vi "REFPROP2dll_Test.vi"(8 "error in (no error)":errorcluster) -> (0 "error out":errorcluster, 3 "Passed?":bool)   [LabVIEW 2016]
panel:
  out "Inputs":T1
  out "Outputs":T2 {"Output" format="%#_9g"}
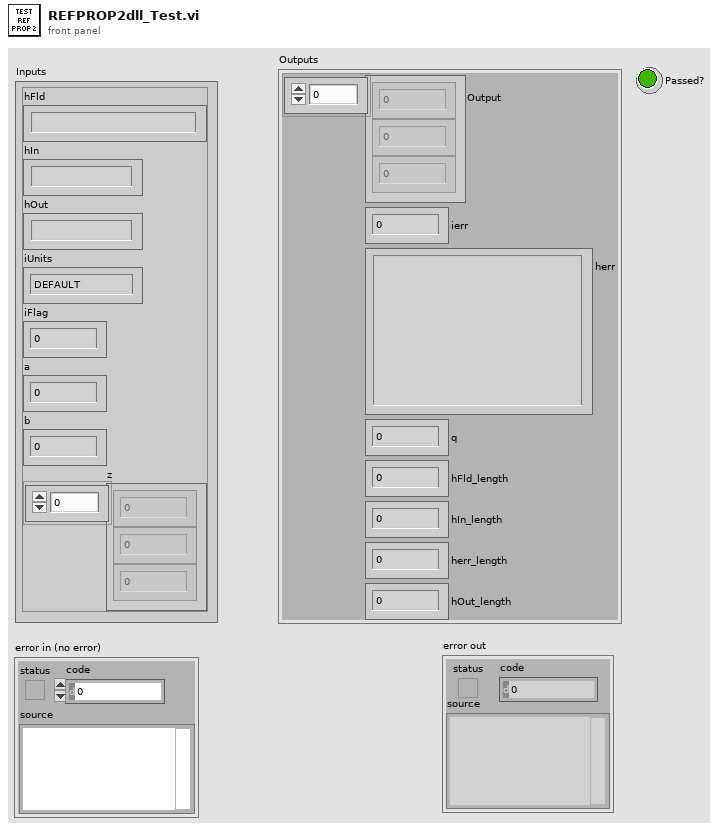
[diagram p1: front panel]
types:
  T1 = cluster{"hFld":string, "hIn":string, "hOut":string, "iUnits":enum32{"DEFAULT", "MOLE SI", "MASS SI", "SI WITH C"}, "iFlag":i32, "a":dbl, "b":dbl, "z":dbl[]}
  T2 = cluster{"Output":dbl[], "ierr":i32, "herr":string, "q":dbl, "hFld_length":i32, "hIn_length":i32, "hOut_length":i32, "herr_length":i32}
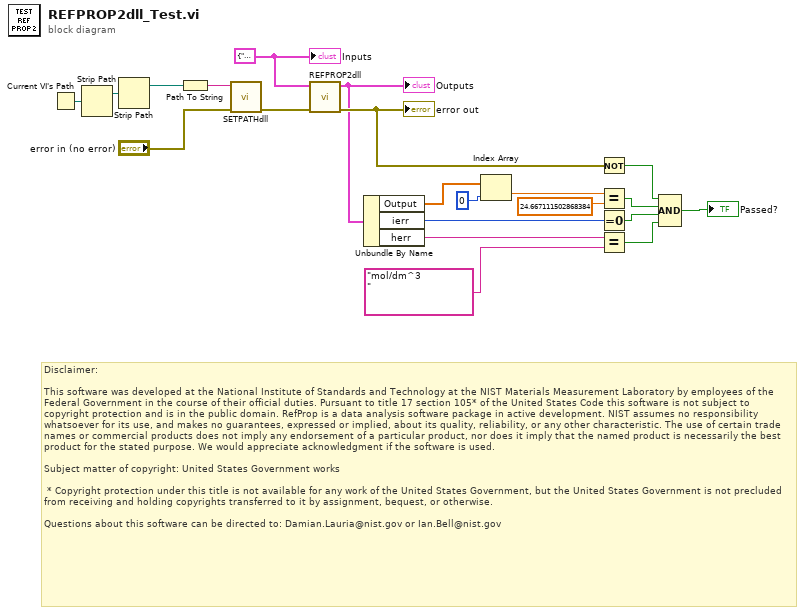
[diagram p0: block diagram]
diagram:
  w16 = T1 {"hFld"="Methane * Ethane", "hIn"="TQ", "hOut"="D", "iUnits"=enum."DEFAULT", "iFlag"=0, "a"=80.0, "b"=0.0, "z"=[0.4, 0.6]} ("Inputs")
  # "Disclaimer:\n\nThis software was developed at the National Institute of Standards and Technology at the NIST Materials Measurement Laboratory by employees of the Federal Government in the course of their official duties. Pursuant to title 17 section 105* of the United States Code this software is not subject to copyright protection and is in the public domain. RefProp is a data analysis software package in active development. NIST assumes no responsibility whatsoever for its use, and makes no guarantees, expressed or implied, about its quality, reliability, or any other characteristic. The use of certain trade names or commercial products does not imply any endorsement of a particular product, nor does it imply that the named product is necessarily the best product for the stated purpose. We would appreciate acknowledgment if the software is used.\n \nSubject matter of copyright: United States Government works\n  \n * Copyright protection under this title is not available for any work of the United States Government, but the United States Government is not precluded from receiving and holding copyrights transferred to it by assignment, bequest, or otherwise.\n\nQuestions about this software can be directed to: Damian.Lauria@nist.gov or Ian.Bell@nist.gov"
  n1 = Current VI's Path() -> (path=w21:path)
  n2 = Strip Path(path=w21) -> (stripped path=w20:path)  [unwired: 1 out]
  n3 = Strip Path(path=w20) -> (stripped path=w19:path)  [unwired: 1 out]
  n4 = Path To String(path=w19) -> (string=w18:string)
  n5 = call "SETPATHdll.vi"("error in (no error)"="error in (no error)", "hpath"=w18) -> ("error out"=w15:errorcluster)  [unwired: 7 in, 2 out]
  n6 = call "REFPROP2dll.vi"("error in (no error)"=w15, "Inputs"=w16) -> ("error out"=w14:errorcluster, "Outputs"=w13:T2)  [unwired: 8 in]
  "error out" <- w14
  "Outputs" <- w13
  n7 = Unbundle By Name(w13) -> ("Output"=w11:dbl[], "ierr"=w12:i32, "herr"=w7:string)
  n8 = Index Array(array=w11, index=0) -> (element=w10:dbl)
  n9 = Not(x=w14) -> (.not. x?=w5:bool)
  n10 = Equal?(x=w10, y=24.667111502868384 ("element")) -> (x = y?=w4:bool)
  n11 = Equal To 0?(x=w12) -> (x = 0?=w3:bool)
  n12 = Equal?(x=w7, y="mol/dm^3                                                                                                                                                                                                                                                      ") -> (x = y?=w2:bool)
  n13 = Compound Arithmetic op=AND(w5, w4, w3, w2) -> (→"Passed?":bool)
  "Inputs" <- w16
